vi "读取excel.vi"(8 "错误输入（无错误）":errorcluster, 10 "路径":path) -> (0 "错误输出":errorcluster, 2 "数据":dbl[][](array[numeric]))   [LabVIEW 2013]
panel:
  in  "数组":dbl[][](array[numeric])
  in  "Excel._Worksheet":refnum<k7>
  in  "Excel._Application":refnum<k7>
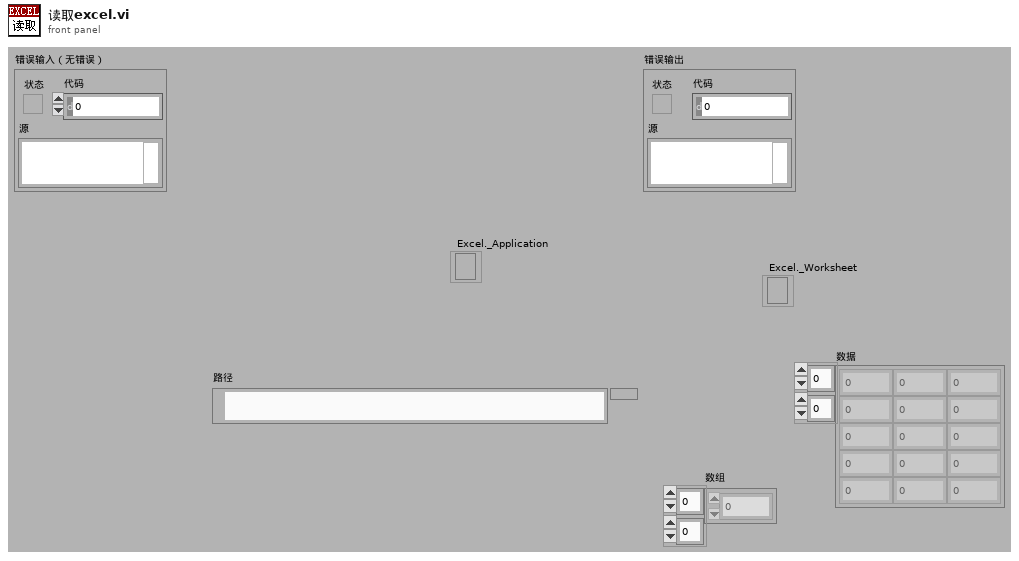
[diagram p1: front panel]
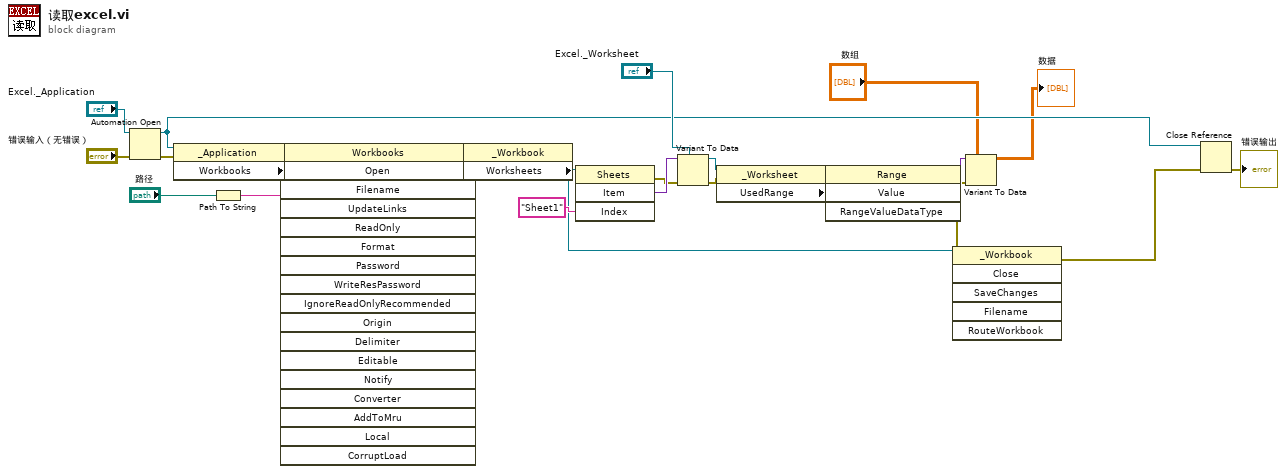
[diagram p0: block diagram]
diagram:
  n1 = Automation Open(error in (no error)="错误输入（无错误）", Automation Refnum="Excel._Application") -> (Automation Refnum=w6:refnum<k7>, error out=w27:errorcluster)  [unwired: 2 out]
  n2 = property class="_Application"(reference=w6, error in=w27) -> (error out=w26:errorcluster, "Workbooks"=w9:refnum<k7>)  [unwired: 1 out]
  n3 = Path To String(path="路径") -> (string=w8:string)
  n4 = invoke class="Workbooks" method="Open"(reference=w9, error in=w26, "Filename"=w8) -> (error out=w24:errorcluster, "Open"=w25:refnum<k7>)  [unwired: 15 in, 16 out]
  n5 = property class="_Workbook"(reference=w25, error in=w24) -> (reference out=w7:refnum<k7>, "Worksheets"=w23:refnum<k7>)  [unwired: 1 out]
  n6 = invoke class="Sheets" method="Item"(reference=w23, "Index"="Sheet1") -> (error out=w20:errorcluster, "Item"=w22:variant)  [unwired: 2 in, 2 out]
  n7 = Variant To Data(error in=w20, type="Excel._Worksheet", Variant=w22) -> (data=w19:refnum<k7>, error out=w16:errorcluster)
  n8 = property class="_Worksheet"(reference=w19, error in=w16) -> (error out=w15:errorcluster, "UsedRange"=w18:refnum<k7>)  [unwired: 1 out]
  n9 = invoke class="Range" method="Value"(reference=w18, error in=w15) -> (error out=w14:errorcluster, "Value"=w17:variant)  [unwired: 2 in, 2 out]
  n10 = Variant To Data(error in=w14, type="数组", Variant=w17) -> (data=→"数据":dbl[][], error out=w4:errorcluster)
  n11 = invoke class="_Workbook" method="Close"(reference=w7, error in=w4) -> (error out=w5:errorcluster)  [unwired: 4 in, 5 out]
  n12 = Close Reference(reference=w6, error in (no error)=w5) -> (error out=→"错误输出":errorcluster)
